vi "Set WD LED.vi"(8 "error in":errorcluster, 9 "Output":bool, 10 "Watchdog Dish Label":T2, 11 "FPGA_MAIN ref in":T1) -> (0 "error out":errorcluster, 3 "FPGA_MAIN ref out":T1)   [LabVIEW 2009]
uses:
  Watchdog Dish Labels.ctl
  TypeDefs/Sensor TypeDefs/FPGA Main ref.ctl
  <vilib>/rvi/interface/nirviReadWriteControl/nirviReadWriteControl.xnode
  FPGA Bitfiles/Q_IGVC_2010.lvproj_FPGA Target_FPGA_MAIN.vi.lvbitx
  <vilib>/Utility/error.llb/Error Cluster From Error Code.vi
  <vilib>/rvi/errors/niLvFpgaAdjustHostInterfaceError.vi
  <vilib>/rvi/interface/common/niFpgaNodeNameForErrorReporting.ctl
  <vilib>/rvi/errors/niLvFpgaWhatHappensToTopLevelVI.ctl
  NiRioSrv.dll
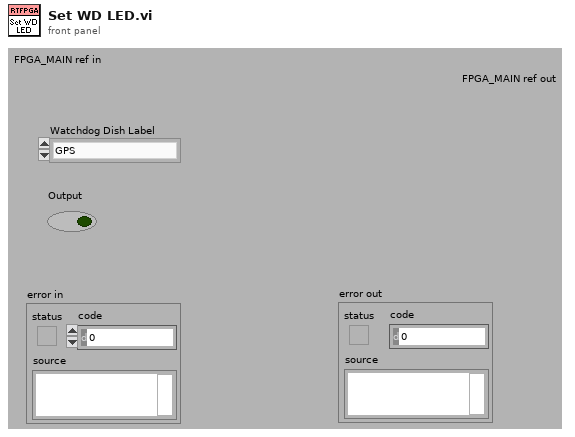
[diagram p1: front panel]
types:
  T1 = typedef "FPGA Main ref.ctl" = refnum<k20>
  T2 = typedef "Watchdog Dish Labels.ctl" = enum16{"GPS", "SICK", "Compass", "Cameras", "Motor Controller", "Debug", "RC Receiver"}
  T3 = typedef "niFpgaNodeNameForErrorReporting.ctl" = enum16{"Open FPGA VI Reference", "Read/Write Control", "Invoke Method: Abort", "Invoke Method: Acknowledge IRQ", "Invoke Method: Download", "Invoke Method: FIFO.Configure", "Invoke Method: FIFO.Read", "Invoke Method: FIFO.Start", "Invoke Method: FIFO.Stop", "Invoke Method: FIFO.Write", "Invoke Method: Reset", "Invoke Method: Run", "Invoke Method: Wait on IRQ", "Close FPGA VI Reference"}
  T4 = typedef "niLvFpgaWhatHappensToTopLevelVI.ctl" = enum16{"top level VI scripted behind XNode", "top level VI inlined behind XNode"}
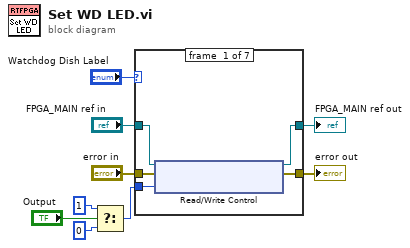
[diagram p0: block diagram]
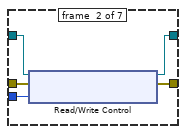
[diagram p2: hidden frame]
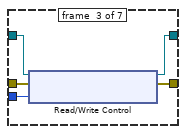
[diagram p3: hidden frame]
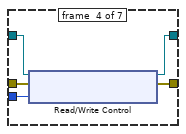
[diagram p4: hidden frame]
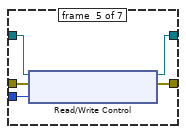
[diagram p5: hidden frame]
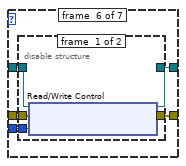
[diagram p6: hidden frame]
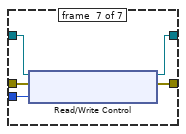
[diagram p8: hidden frame]
diagram:
  n1 = Select(t=u8 1 ("LED1 ON/OFF/BLINK"), s="Output", f=u8 0 ("LED1 ON/OFF/BLINK")) -> (s? t:f=w5:u8)
  n2 = case shown="\"Debug\"" "Watchdog Dish Label" {
    tunnel: "FPGA_MAIN ref in" -> [w14 w54 w96 w137 w178 w219 w267]
    tunnel: w5 -> [w13 w55 w94 w135 w176 w217 w266]
    tunnel: "error in" -> [w12 w53 w95 w136 w177 w218 w265]
    tunnel: [w11 w51 w92 w133 w174 w216 w264] -> w3
    tunnel: [w10 w52 w93 w134 w175 w215 w263] -> w2
    frame #0 {
      n3 = xnode "Read/Write Control"("FPGA VI Reference In"=w14, "error in"=w12, "LED1 ON/OFF/BLINK"=w13) -> ("FPGA VI Reference Out"=w10:T1, "error out"=w11:errorcluster)
    }
    frame #1 {
      n4 = xnode "Read/Write Control"("FPGA VI Reference In"=w54, "error in"=w53, "LED2 ON/OFF/BLINK"=w55) -> ("FPGA VI Reference Out"=w52:T1, "error out"=w51:errorcluster)
    }
    frame #2 {
      n5 = xnode "Read/Write Control"("FPGA VI Reference In"=w96, "error in"=w95, "LED3 ON/OFF/BLINK"=w94) -> ("FPGA VI Reference Out"=w93:T1, "error out"=w92:errorcluster)
    }
    frame #3 {
      n6 = xnode "Read/Write Control"("FPGA VI Reference In"=w137, "error in"=w136, "LED4 ON/OFF/BLINK"=w135) -> ("FPGA VI Reference Out"=w134:T1, "error out"=w133:errorcluster)
    }
    frame #4 {
      n7 = xnode "Read/Write Control"("FPGA VI Reference In"=w178, "error in"=w177, "LED5 ON/OFF/BLINK"=w176) -> ("FPGA VI Reference Out"=w175:T1, "error out"=w174:errorcluster)
    }
    frame #5 {
      n8 = disable-structure shown="Enabled" {
        disable-tunnel: w219 -> [w224 w262]
        disable-tunnel: w218 -> [w223 w261]
        disable-tunnel: w217 -> [w222 _]
        disable-tunnel: [w221 w261] -> w216
        disable-tunnel: [w220 w262] -> w215
        frame #0 {
          n9 = xnode "Read/Write Control"("FPGA VI Reference In"=w224, "error in"=w223, "LED6 ON/OFF/BLINK"=w222) -> ("FPGA VI Reference Out"=w220:T1, "error out"=w221:errorcluster)
        }
        frame #1 {
        }
      }
    }
    frame #6 {
      n10 = xnode "Read/Write Control"("FPGA VI Reference In"=w267, "error in"=w265, "LED7 ON/OFF/BLINK"=w266) -> ("FPGA VI Reference Out"=w263:T1, "error out"=w264:errorcluster)
    }
  }
  "FPGA_MAIN ref out" <- w2
  "error out" <- w3
